vi "GT Set Lead Screw Comp.vi"(0 "cardNum":i16, 1 "lenPos":i32, 2 "pCompNeg":i32, 5 "axis":i16, 7 "n":i16, 9 "startPos":i32, 11 "error in (no error)":errorcluster caption="错误输入（无错误）", 12 "pCompPos":i32) -> (4 "pCompNeg out":i32, 6 "function return":i16, 14 "pCompPos out":i32, 15 "error out":errorcluster caption="错误输出")   [LabVIEW 2020, in "gts.lvlib"]
doc: "GT_API GT_SetLeadScrewComp(short cardNum,short axis,short n,long startPos,long lenPos,long *pCompPos,long *pCompNeg);"
uses:
  gts.lvlib
  dll/32bit/multi_card/gts.dll
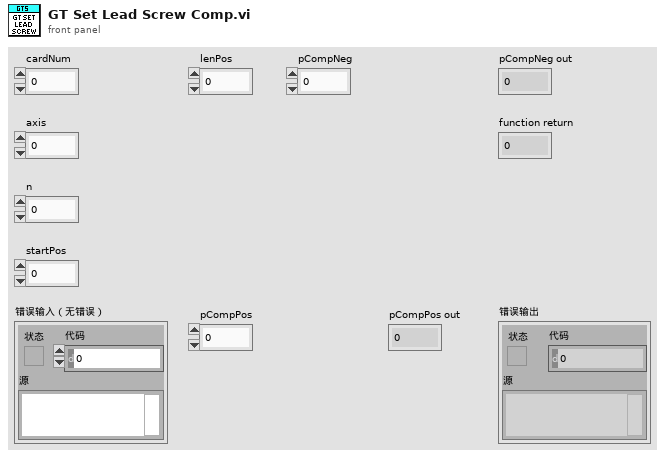
[diagram p1: front panel]
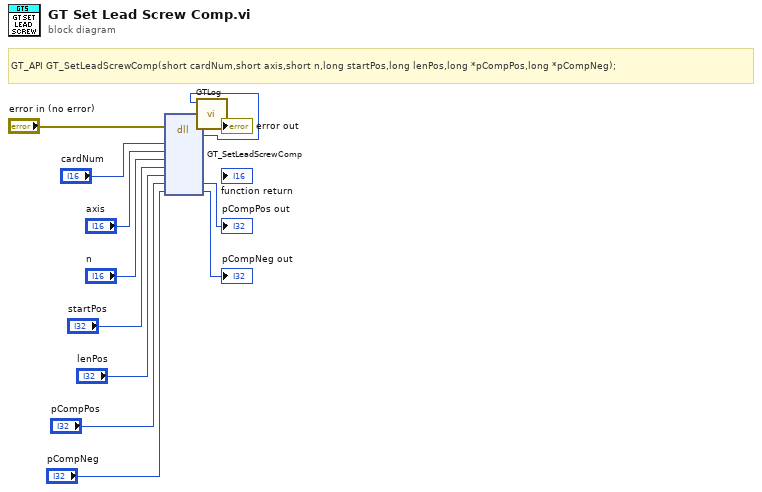
[diagram p0: block diagram]
diagram:
  # "GT_API GT_SetLeadScrewComp(short cardNum,short axis,short n,long startPos,long lenPos,long *pCompPos,long *pCompNeg);"
  n1 = dll-call lib="C:/1228/dll/32bit/multi_card/gts.dll" fn="GT_SetLeadScrewComp"(error in="error in (no error)", "cardNum"="cardNum", "axis"="axis", "n"="n", "startPos"="startPos", "lenPos"="lenPos", "pCompPos"="pCompPos", "pCompNeg"="pCompNeg") -> (error out=w3:errorcluster, w1:i16, "pCompPos"=→"pCompPos out":i32, "pCompNeg"=→"pCompNeg out":i32)  [unwired: 7 in, 1 out]
  n2 = call "GTLog.vi"("error in (no error)"=w3, "Numeric"=w1) -> ("error out"=→"error out":errorcluster)  [unwired: 9 in]
